vi "Parse Sensor Group 2.vi"(11 "stream in":u8[](array[numeric])) -> (1 "Sensor Group 2":T1 {"Infrared" format="%02x"}, 3 "stream out":u8[](array[numeric]))   [LabVIEW 2014]
doc: "Read Sensor Group 2 from a UART data stream."
uses:
  Sensor Group 2.ctl
  Buttons.ctl
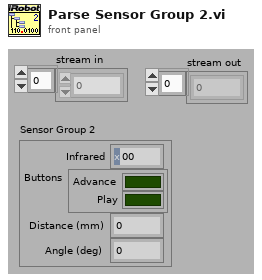
[diagram p1: front panel]
types:
  T1 = typedef "Sensor Group 2.ctl" = cluster{"Infrared":u8, "Buttons":T2, "Distance (mm)":i32, "Angle (deg)":i32}
  T2 = typedef "Buttons.ctl" = cluster{"Advance":bool, "Play":bool}
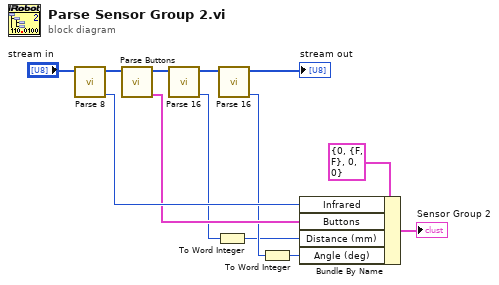
[diagram p0: block diagram]
diagram:
  n1 = call "Parse 8.vi"("stream in"="stream in") -> ("value"=w10:u8, "stream out"=w9:u8[])  [unwired: 9 out]
  n2 = call "Parse Buttons.vi"("stream in"=w9) -> ("Buttons"=w8:T2, "stream out"=w7:u8[])  [unwired: 9 out]
  n3 = call "Parse 16.vi"("stream in"=w7) -> ("value"=w4:u16, "stream out"=w6:u8[])  [unwired: 9 out]
  n4 = To Word Integer(number=w4) -> (16bit integer=w1:i16)
  n5 = call "Parse 16.vi"("stream in"=w6) -> ("value"=w2:u16, "stream out"=→"stream out":u8[])  [unwired: 9 out]
  n6 = To Word Integer(number=w2) -> (16bit integer=w3:i16)
  n7 = Bundle By Name(cluster=T1 {"Infrared"=0, "Buttons"={"Advance"=FALSE, "Play"=FALSE}, "Distance (mm)"=0, "Angle (deg)"=0} ("Sensor Group 2"), "Infrared"=w10, "Buttons"=w8, "Distance (mm)"=w1, "Angle (deg)"=w3) -> (→"Sensor Group 2":T1)
